vi "SpotlightCtrl.vi"(10 "Direction":i16) -> ()   [LabVIEW 2015]
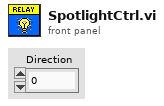
[diagram p1: front panel]
types:
  T1 = typedef "WPI_RelayDevRef.ctl" = cluster{"DevStatus":errorcluster, "Relay Channel":T2, "Relay Direction":T3}
  T2 = typedef "FPGA_DIORelayChannel.ctl" = enum8{"Relay 0", "Relay 1", "Relay 2", "Relay 3", "Invalid"}
  T3 = typedef "WPI_RelayDirection.ctl" = enum16{"Both directions", "Forward only", "Reverse only"}
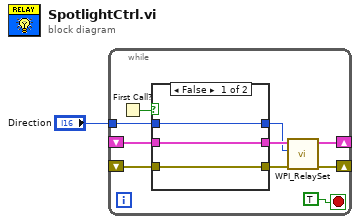
[diagram p0: block diagram]
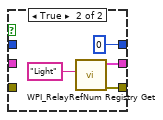
[diagram p2: hidden frame]
diagram:
  n1 = while {
    shift-right: [w8] -> _
    shift-left: _ -> [w5]
    shift-right: [w7] -> _
    shift-left: _ -> [w4]
    tunnel: "Direction" -> [w2]
    stop <- TRUE stop-if-true
    n2 = First Call?() -> (First Call?: T/F=w11:bool)
    n3 = case shown="False" w11 {
      tunnel: [w14 w17] -> w10
      tunnel: [w13 w16] -> w9
      tunnel: w5 -> [w14 _]
      tunnel: w4 -> [w13 _]
      tunnel: [w12 i16 0 ("Direction")] -> w3
      tunnel: w2 -> [w12 _]
      frame False {
      }
      frame True {
        n4 = call <vilib>:"WPI_RelayRefNum Registry Get.vi"("refnum name"="Light") -> ("error out"=w16:errorcluster, "RelayDevRef"=w17:T1)  [unwired: 9 in]
      }
    }
    n5 = call <vilib>:"WPI_RelaySet.vi"("error in (no error)"=w9, "RelayValue"=w3, "RelayDevRef"=w10) -> ("error out"=w7:errorcluster, "RelayDevRef"=w8:T1)  [unwired: 7 in]
  }
